vi "Configure Trigger Advanced.vi"(8 "error in (no error)":errorcluster, 9 "Trigger Level (3.3 V)":dbl=3.3, 10 "Channel (1: 1)":i32(ring)=1 items=["1"=1, "2"=2], 11 "VISA resource name":refnum<visa-resource-name>) -> (0 "error out":errorcluster, 3 "VISA resource name out":refnum<visa-resource-name>)   [LabVIEW 2026, in "Agilent 3352X Series.lvlib"]
doc: "Configures the output trigger level and input trigger threshold in volts.\n\n<B>Note</B>: \n(1) This VI is only applicable for 33611A, 33612A, 33621A and 33622A models.\n(2) This VI does not check the instrument status."
uses:
  Agilent 3352X Series.lvlib
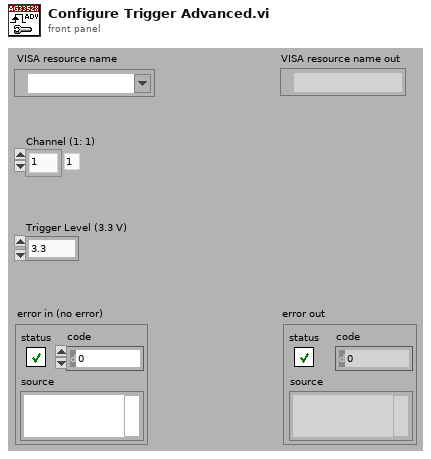
[diagram p1: front panel]
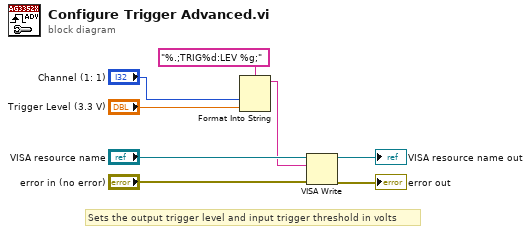
[diagram p0: block diagram]
diagram:
  # "Sets the output trigger level and input trigger threshold in volts"
  n1 = Format Into String(format string="%.;TRIG%d:LEV %g;", "Channel (1: 1)", "Trigger Level (3.3 V)") -> (resulting string=w1:string)  [unwired: 2 in, 1 out]
  n2 = VISA Write(VISA resource name="VISA resource name", write buffer=w1, error in (no error)="error in (no error)") -> (VISA resource name out=→"VISA resource name out":refnum<visa-resource-name>, error out=→"error out":errorcluster)  [unwired: 1 out]
